vi "calculate #pixels.vi"(8 "error in (no error)":errorcluster, 11 "Simulated Camera in":refnum<class "Sim_Ixon_Ultra.lvclass">) -> (0 "error out":errorcluster, 2 "#pixels":dbl, 3 "Simulated Camera out":refnum<class "Sim_Ixon_Ultra.lvclass">)   [LabVIEW 2018]
uses:
  Sim_Ixon_Ultra.lvclass
  C:/Users/Denis/Desktop/S4ACS/S4ACS/Simulated_CCD_Camera/Simulated Camera.lvclass
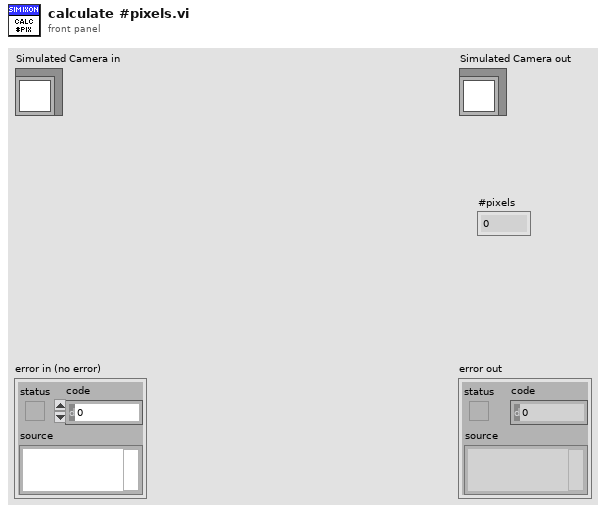
[diagram p1: front panel]
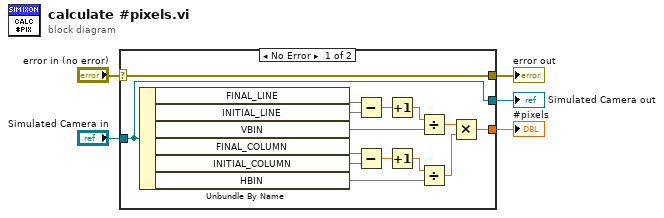
[diagram p0: block diagram]
diagram:
  n1 = case shown="No Error" "error in (no error)" {
    selector: "error in (no error)" -> [w20 w22]
    tunnel: [w20 w22] -> w4
    tunnel: [w19 w21] -> w2
    tunnel: "Simulated Camera in" -> [w19 w21]
    tunnel: [w6 _] -> w1
    frame No Error {
      n2 = Unbundle By Name(w19) -> ("FINAL_LINE"=w18, "INITIAL_LINE"=w17, "VBIN"=w11, "FINAL_COLUMN"=w16, "INITIAL_COLUMN"=w15, "HBIN"=w9)
      n3 = Subtract(x=w18, y=w17) -> (x-y=w14:dbl)
      n4 = Subtract(x=w16, y=w15) -> (x-y=w13:dbl)
      n5 = Increment(x=w14) -> (x+1=w12:dbl)
      n6 = Increment(x=w13) -> (x+1=w10:dbl)
      n7 = Divide(x=w12, y=w11) -> (x/y=w8:dbl)
      n8 = Divide(x=w10, y=w9) -> (x/y=w7:dbl)
      n9 = Multiply(x=w8, y=w7) -> (x*y=w6:dbl)
    }
    frame Error {
    }
  }
  "error out" <- w4
  "Simulated Camera out" <- w2
  "#pixels" <- w1
